vi "IPS120 WH0 - Send Command.vi"(1 "Command String":string, 2 "GPIB Address":string) -> (0 "Response String":string)   [LabVIEW 2009]
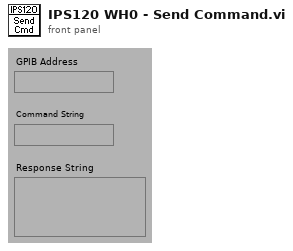
[diagram p1: front panel]
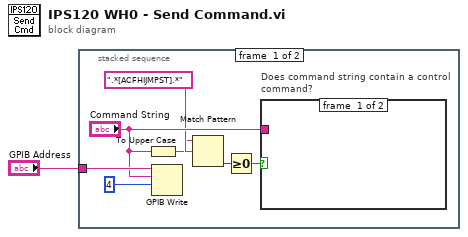
[diagram p0: block diagram]
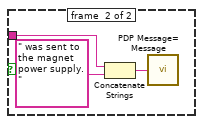
[diagram p2: hidden frame]
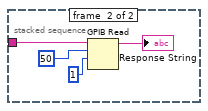
[diagram p3: hidden frame]
diagram:
  n1 = stacked-sequence {
    tunnel: "GPIB Address" -> [w7 w13]
    frame #0 {
      n2 = To Upper Case(1:"Command String") -> (0:w4:string)
      n3 = GPIB Write(0:w7, 1:"Command String", 2:i16 4 ("mode (0)")) -> ()  [unwired: 2 in, 2 out]
      n4 = Match Pattern(string=w4, regular expression=".*[ACFHIJMPST].*") -> (offset past match=w2:i32)  [unwired: 1 in, 3 out]
      n5 = Greater Or Equal To 0?(x=w2) -> (x >= 0?=w3:bool)
      n6 = case "Does command string contain a control command?" shown="True" w3 {
        tunnel: "Command String" -> [_ w11]
        frame #0 {
        }
        frame #1 {
          n7 = Concatenate Strings(w11, " was sent to the magnet power supply.") -> (w9:string)
          n8 = call "PDP Message= Message.vi"("Message"=w9) -> ()
        }
      }
    }
    frame #1 {
      n9 = GPIB Read(0:w13, 1:50 ("byte count"), 2:i16 1 ("mode (0)")) -> (5:→"Response String":string)  [unwired: 2 in, 2 out]
    }
  }
